vi "Load_Config.vi"(8 "Error In":errorcluster, 11 "Data":T2={"Info Box"="", "MAC & Name Out"=[], "Default Gateway"="", "Drfiter IP Addresses"=[], "Network Map"="", "Drifter Selection"=0, "File Selection"=0, "Download File Path"=path "", "File Selection Strings"=[], "Sample Rate"=enum." 0.2", "Log While Charging"=enum." Yes"}) -> (0 "Error Out":errorcluster, 1 "Log While\nCharging":enum32{"No Selection", " Yes", " No"}(radio) caption="Radio Buttons", 2 "Sample\nRate":T1(radio) caption="Radio Buttons", 3 "File Contents":string)   [LabVIEW 2017]
uses:
  data.ctl
panel:
  out "trimmed string":string
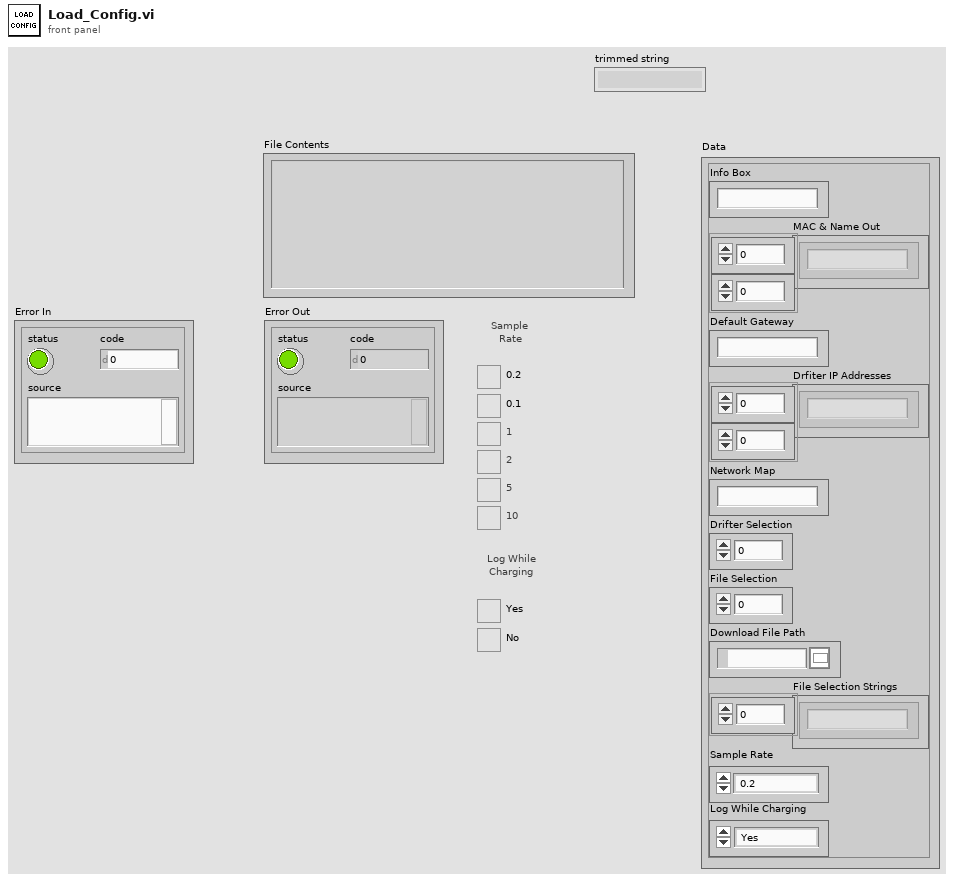
[diagram p1: front panel]
types:
  T1 = enum32{"No Selection", " 0.2", " 0.1", " 1", " 2", " 5", " 10"}
  T2 = typedef "data.ctl" = cluster{"Info Box":string, "MAC & Name Out":string[][], "Default Gateway":string, "Drfiter IP Addresses":string[][], "Network Map":string, "Drifter Selection":i32, "File Selection":i32, "Download File Path":path, "File Selection Strings":string[], "Sample Rate":enum32{"No Selection", " 0.2", " 0.1", " 1", " 2", " 5", " 10"}, "Log While Charging":enum32{"No Selection", " Yes", " No"}}
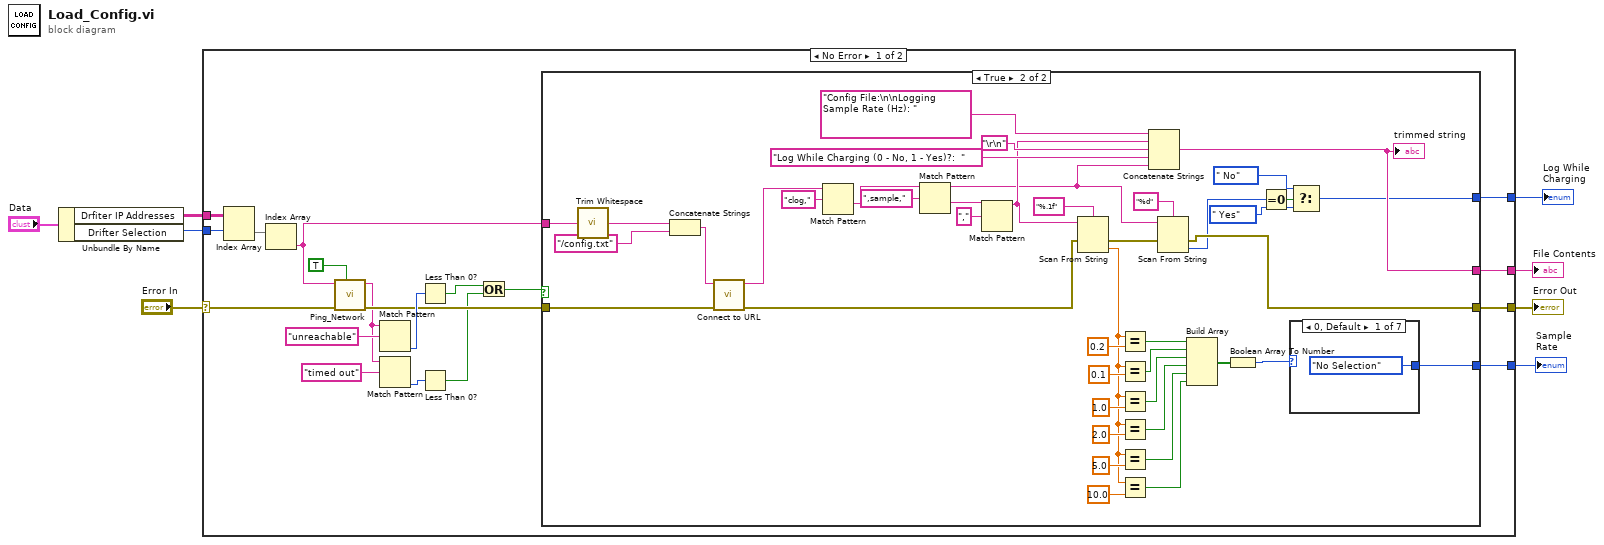
[diagram p0: block diagram]
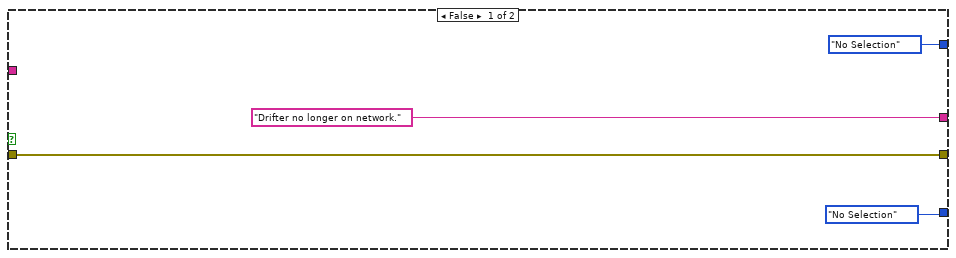
[diagram p2: hidden frame]
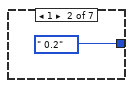
[diagram p3: hidden frame]
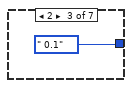
[diagram p4: hidden frame]
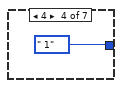
[diagram p5: hidden frame]
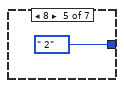
[diagram p6: hidden frame]
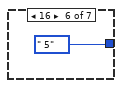
[diagram p7: hidden frame]
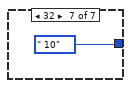
[diagram p8: hidden frame]
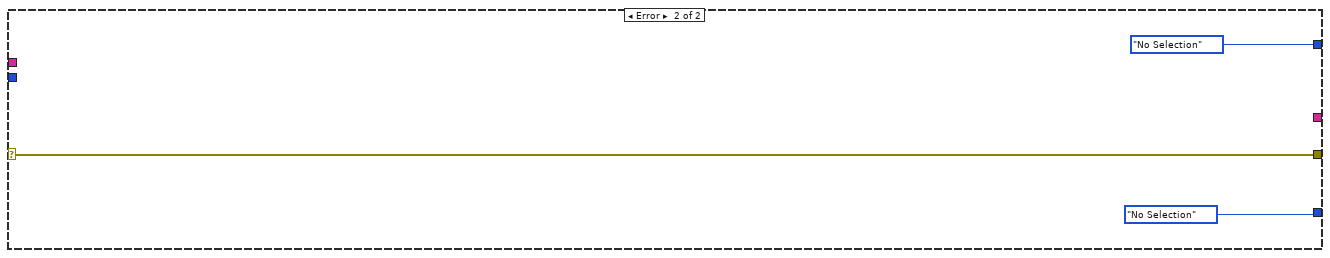
[diagram p9: hidden frame]
diagram:
  n1 = Unbundle By Name("Data") -> ("Drfiter IP Addresses"=w6:string[][], "Drifter Selection"=w5:i32)
  n2 = case shown="No Error" "Error In" {
    selector: "Error In" -> [w19 w84]
    tunnel: [w27 w84] -> w7
    tunnel: w6 -> [w21 _]
    tunnel: w5 -> [w18 _]
    tunnel: [w17 _] -> w3
    tunnel: [w16 enum32{"No Selection", " Yes", " No"}."No Selection" ("Log While\nCharging")] -> w2
    tunnel: [w15 T1."No Selection" ("Sample\nRate")] -> w1
    frame No Error {
      n3 = Index Array(array=w21, index (row)=w18) -> (element=w26:string[])  [unwired: 1 in]
      n4 = Index Array(array=w26) -> (element=w20:string)  [unwired: 1 in]
      n5 = call "Ping_Network.vi"("IP/Default Gateway (T/F)"=TRUE, "Error In"=w19, "Default Gateway/IP"=w20) -> ("Error Out"=w22:errorcluster, "Terminal Output"=w14:string)  [unwired: 7 in]
      n6 = Match Pattern(string=w14, regular expression="unreachable") -> (offset past match=w23:i32)  [unwired: 1 in, 3 out]
      n7 = Match Pattern(string=w14, regular expression="timed out") -> (offset past match=w10:i32)  [unwired: 1 in, 3 out]
      n8 = Less Than 0?(x=w23) -> (x < 0?=w11:bool)
      n9 = Less Than 0?(x=w10) -> (x < 0?=w9:bool)
      n10 = Or(x=w11, y=w9) -> (x .or. y?=w12:bool)
      n11 = case shown="True" w12 {
        tunnel: w22 -> [w31 w74]
        tunnel: [w31 w59] -> w27
        tunnel: w20 -> [_ w70]
        tunnel: ["Drifter no longer on network." ("Body") w64] -> w17
        tunnel: [enum32{"No Selection", " Yes", " No"}."No Selection" ("Log While\nCharging") w50] -> w16
        tunnel: [T1."No Selection" ("Sample\nRate") w32] -> w15
        frame False {
        }
        frame True {
          n12 = call <vilib>:"Trim Whitespace.vi"("string"=w70) -> ("trimmed string"=w73:string)  [unwired: 1 in]
          n13 = Concatenate Strings(w73, "/config.txt" ("string")) -> (w71:string)
          n14 = call "Connect to URL.vi"("Error In"=w74, "URL"=w71) -> ("Error Out"=w61:errorcluster, "Body"=w68:string)  [unwired: 8 in]
          n15 = Match Pattern(string=w68, regular expression="clog,") -> (after substring=w66:string)  [unwired: 1 in, 3 out]
          n16 = Match Pattern(string=w66, regular expression=",sample,") -> (before substring=w48:string, after substring=w57:string)  [unwired: 1 in, 2 out]
          n17 = Match Pattern(string=w57, regular expression=",") -> (before substring=w49:string)  [unwired: 1 in, 3 out]
          n18 = Scan From String(format string="%.1f", input string=w49, error in=w61) -> (error out=w60:errorcluster, output 1=w33:dbl)  [unwired: 2 in, 2 out]
          n19 = Equal?(x=w33, y=0.2) -> (x = y?=w47:bool)
          n20 = Equal?(x=w33, y=0.1) -> (x = y?=w46:bool)
          n21 = Equal?(x=w33, y=1.0) -> (x = y?=w45:bool)
          n22 = Equal?(x=w33, y=2.0) -> (x = y?=w44:bool)
          n23 = Equal?(x=w33, y=5.0) -> (x = y?=w43:bool)
          n24 = Equal?(x=w33, y=10.0) -> (x = y?=w42:bool)
          n25 = Concatenate Strings("Config File:\n\nLogging Sample Rate (Hz): ", w49, "\r\n", "Log While Charging (0 - No, 1 - Yes)?:  ", w48) -> (w64:string)
          "trimmed string" <- w64
          n26 = Scan From String(format string="%d", input string=w48, error in=w60) -> (error out=w59:errorcluster, output 1=w53:i32)  [unwired: 2 in, 2 out]
          n27 = Build Array(w47, w46, w45, w44, w43, w42) -> (w41:bool[])
          n28 = Boolean Array To Number(Boolean array=w41) -> (number=w40:u32)
          n29 = Equal To 0?(x=w53) -> (x = 0?=w54:bool)
          n30 = case shown="0, Default" w40 {
            tunnel: [T1."No Selection" ("Sample\nRate") T1." 0.2" ("Sample\nRate") T1." 0.1" ("Sample\nRate") T1." 1" ("Sample\nRate") T1." 2" ("Sample\nRate") T1." 5" ("Sample\nRate") T1." 10" ("Sample\nRate")] -> w32
            frame 0, Default {
            }
            frame 1 {
            }
            frame 2 {
            }
            frame 4 {
            }
            frame 8 {
            }
            frame 16 {
            }
            frame 32 {
            }
          }
          n31 = Select(t=enum32{"No Selection", " Yes", " No"}." No" ("Log While\nCharging"), s=w54, f=enum32{"No Selection", " Yes", " No"}." Yes" ("Log While\nCharging")) -> (s? t:f=w50:enum32{"No Selection", " Yes", " No"})
        }
      }
    }
    frame Error {
    }
  }
  "Sample\nRate" <- w1
  "Error Out" <- w7
  "File Contents" <- w3
  "Log While\nCharging" <- w2
